vi "clear buffer array separately.vi"(8 "error in (no error)":errorcluster, 10 "Image array":T1[][](array[typedef]), 11 "ptr array":u64[](array[numeric])) -> (0 "error out":errorcluster)   [LabVIEW 2021, in "Camera.lvlib" / "Camera.lvclass"]
uses:
  Camera.lvclass
  <vilib>/vision/Image Controls.llb/IMAQ Image.ctl
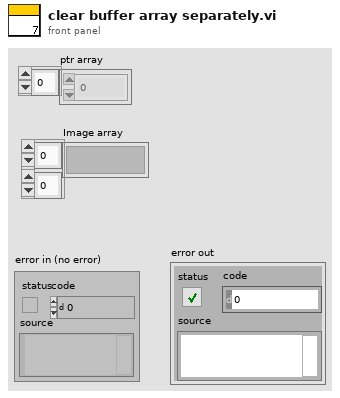
[diagram p1: front panel]
types:
  T1 = typedef "IMAQ Image.ctl" = refnum<image>
  T2 = enum32{"Map Pixel Pointer", "Unmap Pixel Pointer", "Get Pixels Infos"}
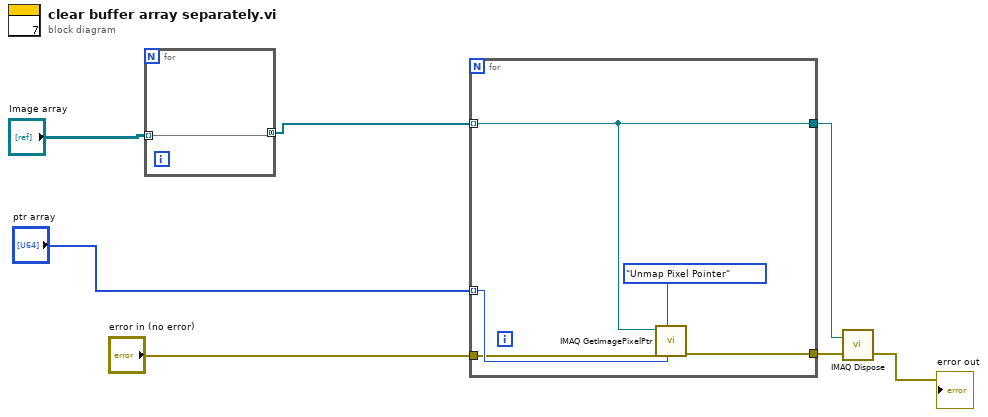
[diagram p0: block diagram]
diagram:
  n1 = for {
    tunnel: "Image array" -> [w8] mode=indexing
    tunnel: [w8] -> w1 mode=concatenating
  }
  n2 = for {
    tunnel: [w10] -> w3
    tunnel: "ptr array" -> [w12] mode=indexing
    tunnel: w1 -> [w9] mode=indexing
    tunnel: "error in (no error)" -> [w11]
    tunnel: [w9] -> w4
    n3 = call "IMAQ GetImagePixelPtr"("Pixel Pointer in"=w12, "Function"=T2."Unmap Pixel Pointer", "error in (no error)"=w11, "Image"=w9) -> ("error out"=w10:errorcluster)  [unwired: 2 in, 5 out]
  }
  n4 = call "IMAQ Dispose"("Image"=w4, "error in (no error)"=w3) -> ("error out"=→"error out":errorcluster)  [unwired: 4 in]
